vi "期末11-3-2.vi"() -> ()   [LabVIEW 2014]
uses:
  <vilib>/vision/NI_Vision_Development_Module.lvlib
panel:
  in  "計數器":dbl
  out "座標和":dbl
  in  "Boolean":bool
  out "Image Out 2":T1(plugin-control)
  out "ROI":T2
  in  "紀錄中點座標和":bool
  out "填入飽和磁場分量尖點座標和 2":dbl
  in  "3. Number of Erosion":i32=10
  out "Image Out":T1(plugin-control)
  in  "紀錄電流":dbl[](array[numeric])
  in  "Tab Control 2":enum32{"座標", "座標和", "作圖"}(tab)
  out "相減結果":dbl[](array[numeric])
  out "尖點座標和":dbl[](array[numeric])
  out "分量-電流":cluster{"紀錄電流":dbl[], dbl[]}(graph)
  in  "結束實驗":bool
  in  "1. 範圍選擇":T3={"色相（H）"={0, 255}, "飽和度（S）"={0, 255}, "亮度（L）"={0, 255}} {"亮度（L）" scale=0.0..255.0; "飽和度（S）" scale=0.0..255.0; "色相（H）" scale=0.0..255.0}
  out "Number of Particles":i32
  out "output cluster":cluster{"X":dbl, "Y":dbl}
  in  "Tab Control":T4(tab)
  out "1. 顏色選取":T1(plugin-control)
  out "2. 填補空隙":T1(plugin-control)
  out "3. 移除雜點":T1(plugin-control)
  out "4. 形狀修正":T1(plugin-control)
  out "5. 選取結果":T1(plugin-control)
  out "Particle Measurements":dbl[][](array[numeric])
  out "Error Out":errorcluster
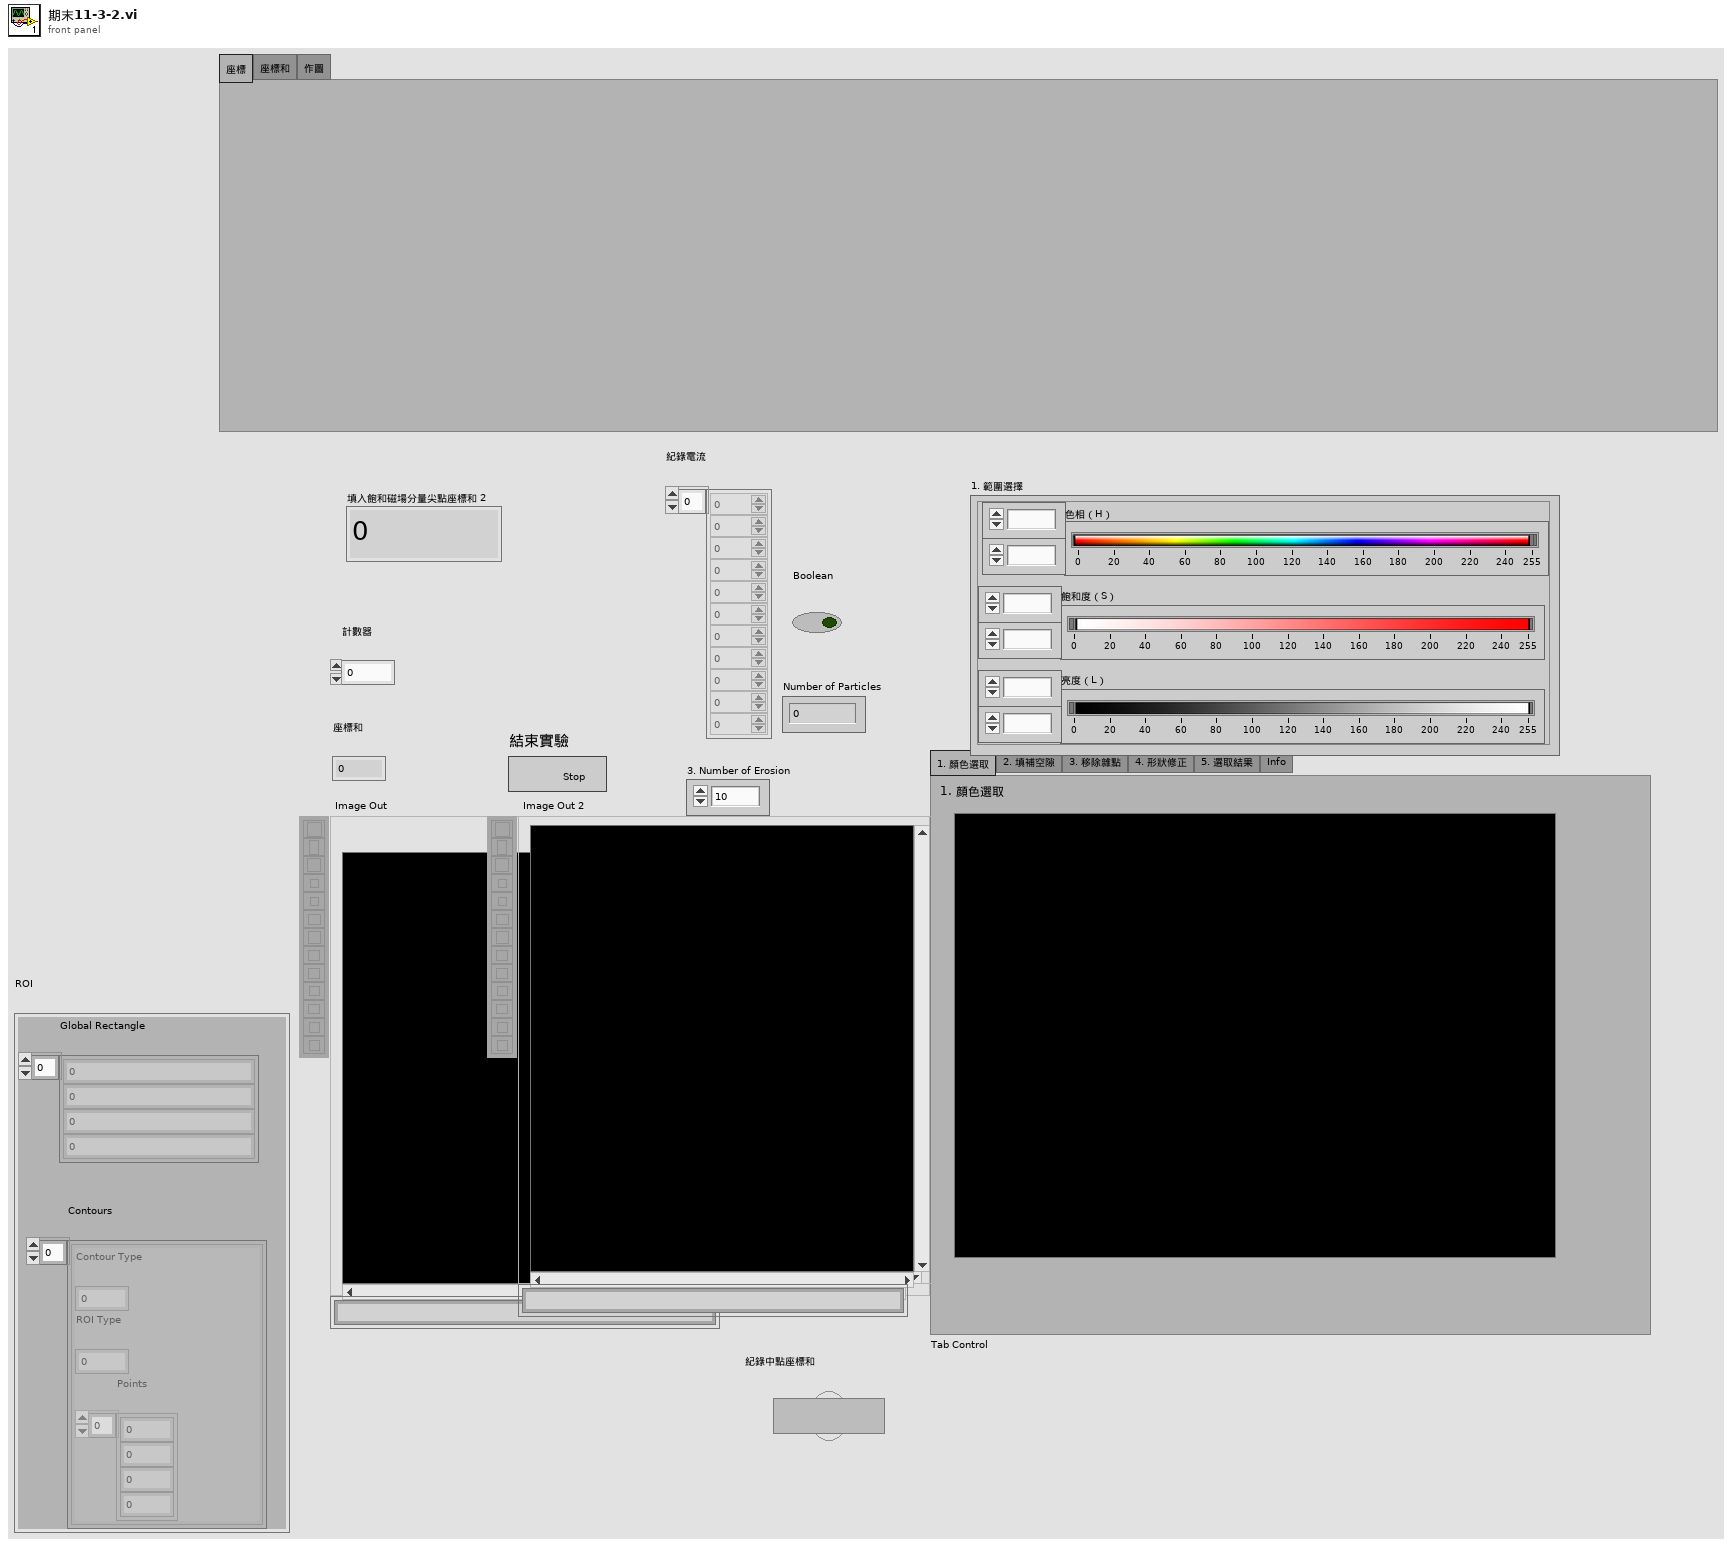
[diagram p1: front panel]
types:
  T1 = typedef "IMAQ Image.ctl" = refnum<image>
  T2 = cluster{"Global Rectangle":i32[], "Contours":cluster{"Contour Type":u32, "ROI Type":u32, "Points":i32[]}[]}
  T3 = cluster{"色相（H）":cluster{u8, u8}, "飽和度（S）":cluster{u8, u8}, "亮度（L）":cluster{u8, u8}}
  T4 = enum32{"1. 顏色選取", "2. 填補空隙", "3. 移除雜點", "4. 形狀修正", "5. 選取結果", "Info"}
  T5 = typedef "Image Type" = u32
  T6 = cluster{"Numeric":dbl, "Numeric":dbl, "Numeric":dbl, "Numeric":dbl}
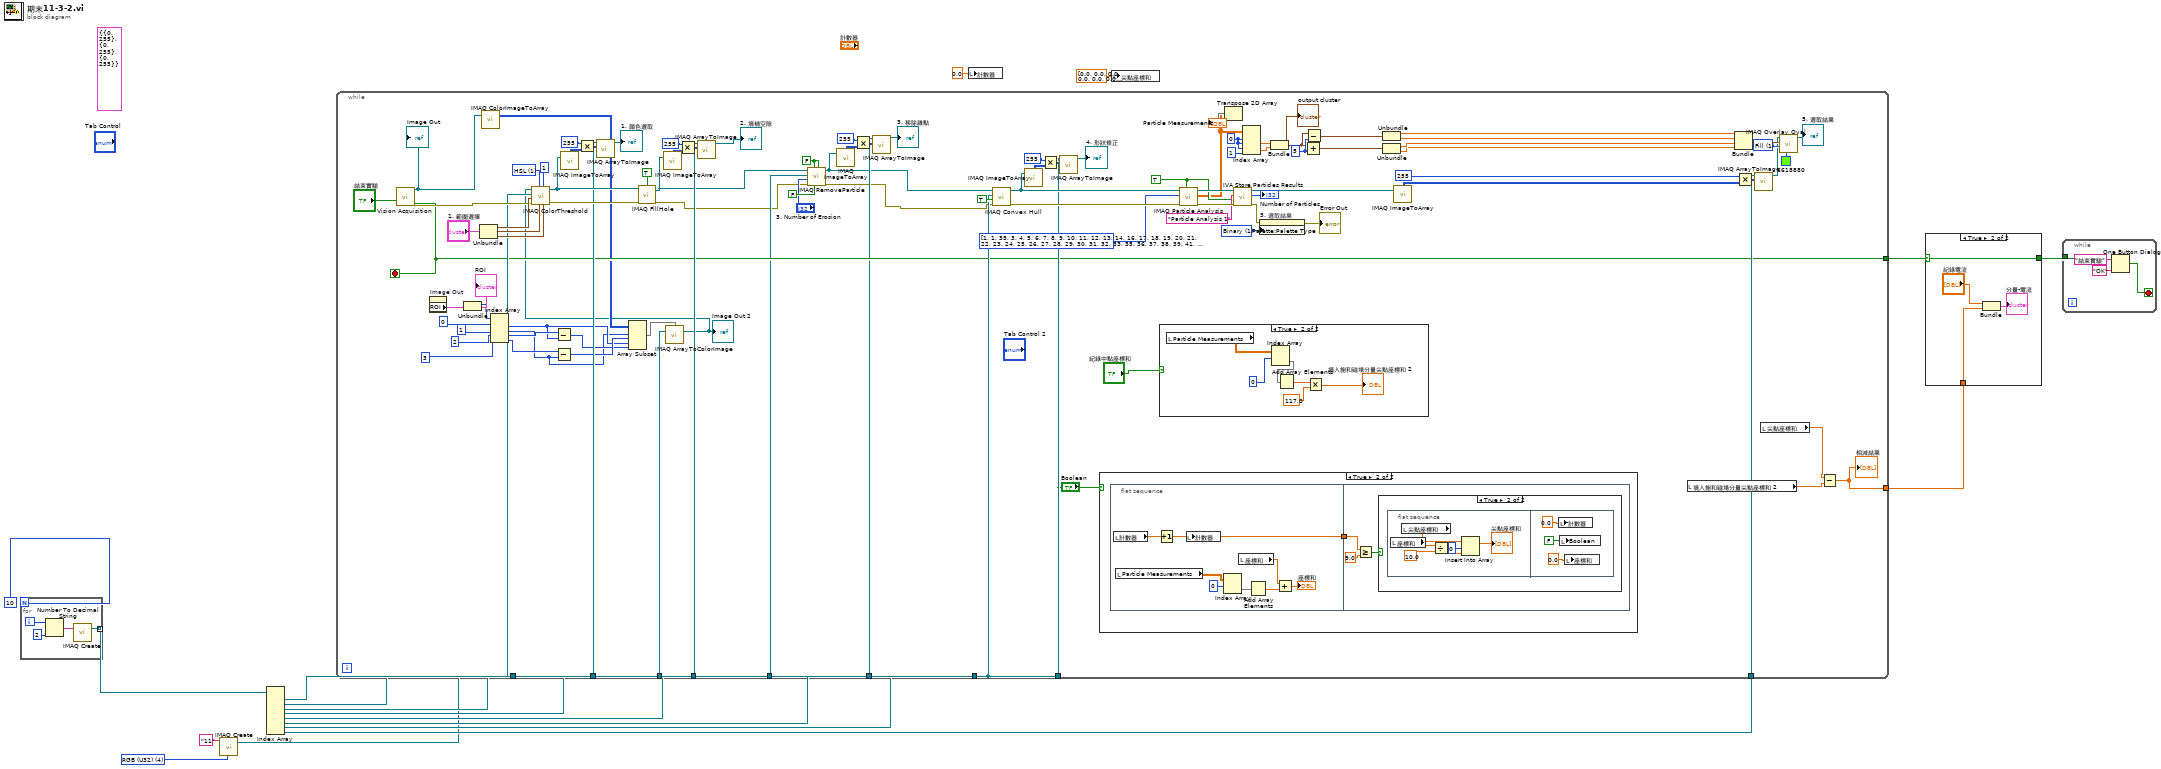
[diagram p0: block diagram]
diagram:
  w5 = T5 4 items=["Grayscale (U8)", "Grayscale (I16)", "Grayscale (SGL)", "Complex (CSG)", "RGB (U32)", "HSL (U32)", "RGB (U64)", "Grayscale (U16)"] ("Image Type")
  (unwired) T3 {"色相（H）"={0, 255}, "飽和度（S）"={0, 255}, "亮度（L）"={0, 255}} ("範圍選擇")
  n1 = for {
    N: 10 -> [_]
    tunnel: [w19] -> w18 mode=indexing
    i -> [w21]
    n2 = Number To Decimal String(number=w21, width (-)=2) -> (decimal integer string=w20:string)
    n3 = call "IMAQ Create"("Image Name"=w20) -> ("New Image"=w19:T1)  [unwired: 4 in, 1 out]
  }
  n4 = call "IMAQ Create"("Image Name"="11", "Image Type"=w5) -> ("New Image"=w6:T1)  [unwired: 3 in, 1 out]
  n5 = Index Array(array=w18) -> (element #1=w17:T1, element #2=w16:T1, element #3=w15:T1, element #4=w8:T1, element #5=w7:T1, element #6=w13:T1, element #7=w12:T1, element #8=w11:T1)  [unwired: 8 in]
  n6 = while {
    tunnel: w15 -> [w92]
    tunnel: w13 -> [w103]
    tunnel: [w103] -> _
    tunnel: w16 -> [w97]
    tunnel: w17 -> [w91]
    tunnel: w12 -> [w85]
    tunnel: w11 -> [w62]
    tunnel: [w58] -> w10
    tunnel: [w26] -> w9
    tunnel: w8 -> [w51]
    tunnel: w7 -> [w50]
    tunnel: w6 -> [w36]
    stop <- w58 stop-if-true
    w55 = FALSE ("Connectivity 4/8 (8)")
    w67 = u32 1 items=["Frame", "Fill"] ("Drawing Mode (Frame)")
    w76 = 5
    w81 = 0
    w105 = u32 1 items=["Grayscale", "Binary", "Gradient", "Rainbow", "Temperature", "User Defined"] ("Palette")
    w110 = i32[] [1, 1, 35, 3, 4, 5, 6, 7, 8, 9, 10, 11, 12, 13, 14, 16, 17, 18, 19, 20, 21, 22, 23, 24, 25, 26, 27, 28, 29, 30, 31, 32, 33, 35, 36, 37, 38, 39, 41, 42, 43, 45, 46, 48, 49, 50, 51, 53, 54, 55, 56, 58, 59, 60, 61, 62, 63, 64, 65, 66, 68, 69, 70, 71, 72, 73, 74, 75, 76, 77, 78, 79, 80, 81, 82, 83, 84, 85, 86, 87, 88] items=["Center of Mass X", "Center of Mass Y", "First Pixel X", "First Pixel Y", "Bounding Rect Left", "Bounding Rect Top", "Bounding Rect Right", "Bounding Rect Bottom", "Max Feret Diameter Start X", "Max Feret Diameter Start Y", "Max Feret Diameter End X", "Max Feret Diameter End Y", "Max Horiz. Segment Length Left", "Max Horiz. Segment Length Right", "Max Horiz. Segment Length Row", "-", "Bounding Rect Width", "Bounding Rect Height", "Bounding Rect Diagonal", "Perimeter", "Convex Hull Perimeter", "Holes' Perimeter", "Max Feret Diameter", "Equivalent Ellipse Major Axis", "Equivalent Ellipse Minor Axis", "Equivalent Ellipse Minor Axis (Feret)", "Equivalent Rect Long Side", "Equivalent Rect Short Side", "Equivalent Rect Diagonal", "Equivalent Rect Short Side (Feret)", "Average Horiz. Segment Length", "Average Vert. Segment Length", "Hydraulic Radius", "Waddel Disk Diameter", "-", "Area", "Holes' Area", "Particle & Holes' Area", "Convex Hull Area", "Image Area", "-", "Number of Holes", "Number of Horiz. Segments", "Number of Vert. Segments", "-", "Orientation", "Max Feret Diameter Orientation", "-", "% Area/Image Area", "% Area/(Particle & Holes' Area)", "Ratio of Equivalent Ellipse Axes", "Ratio of Equivalent Rect Sides", "-", "Elongation Factor", "Compactness Factor", "Heywood Circularity Factor", "Type Factor", "-", "Sum X", "Sum Y", "Sum XX", "Sum XY", "Sum YY", "Sum XXX", "Sum XXY", "Sum XYY", "Sum YYY", "-", "Moment of Inertia XX", "Moment of Inertia XY", "Moment of Inertia YY", "Moment of Inertia XXX", "Moment of Inertia XXY", "Moment of Inertia XYY", "Moment of Inertia YYY", "Norm. Moment of Inertia XX", "Norm. Moment of Inertia XY", "Norm. Moment of Inertia YY", "Norm. Moment of Inertia XXX", "Norm. Moment of Inertia XXY", "Norm. Moment of Inertia XYY", "Norm. Moment of Inertia YYY", "Hu Moment 1", "Hu Moment 2", "Hu Moment 3", "Hu Moment 4", "Hu Moment 5", "Hu Moment 6", "Hu Moment 7"] ("Pixel Measurements")
    w112 = TRUE ("Connectivity 4/8 (8)")
    w121 = u16 1 items=["RGB", "HSL", "HSV", "HSI"] ("Color Mode")
    n7 = call "Vision Acquisition"("Stop (F)"="結束實驗") -> ("Image Out"=w44:T1, "Stopped"=w58:bool, "error out"=w116:errorcluster)  [unwired: 24 in]
    "Image Out" <- w44
    n8 = property on="Image Out" class="ImageControl"() -> ("ROI"=w42:T2)  [unwired: 2 in, 2 out]
    "ROI" <- w42
    n9 = Unbundle(w42) -> ("Global Rectangle"=w41:i32[])  [unwired: 1 out]
    n10 = Unbundle("1. 範圍選擇") -> ("色相（H）"=w120:cluster{u8, u8}, "飽和度（S）"=w119:cluster{u8, u8}, "亮度（L）"=w118:cluster{u8, u8})
    n11 = call "IMAQ ColorImageToArray"("Image"=w44) -> ("Image Pixels (U32)"=w43:u32[][])  [unwired: 3 in, 2 out]
    n12 = Index Array(array=w41, index #1=0 ("index"), index #2=1 ("index"), index #3=2 ("index"), index #4=3 ("index")) -> (element #1=w31:i32, element #2=w29:i32, element #3=w34:i32, element #4=w30:i32)
    n13 = Subtract(x=w34, y=w31) -> (x-y=w32:i32)
    n14 = Subtract(x=w30, y=w29) -> (x-y=w33:i32)
    n15 = Array Subset(array=w43, index (row)=w29, length (row)=w33, index (col)=w31, length (col)=w32) -> (w35:u32[][])
    n16 = call "IMAQ ArrayToColorImage"("Image Pixels (U32)"=w35, "Image"=w36) -> ("Image Out"=w28:T1)  [unwired: 3 in, 1 out]
    "Image Out 2" <- w28
    n17 = call "IMAQ ColorThreshold"("Blue or Luma or Val or Inten Range"=w118, "Replace Value"=1, "Green or Sat Range"=w119, "Color Mode"=w121, "error in (no error)"=w116, "Red or Hue Range"=w120, "Image Dst"=w91, "Image Src"=w28) -> ("error out"=w107:errorcluster, "Image Dst Out"=w102:T1)  [unwired: 2 out]
    n18 = call "IMAQ ImageToArray"("Image"=w102) -> ("Image Pixels (U8)"=w100:u8[][])  [unwired: 3 in, 4 out]
    n19 = Multiply(x=255, y=w100) -> (x*y=w99:i32[][])
    n20 = call "IMAQ ArrayToImage"("Image Pixels (U8)"=w99, "Image"=w97) -> ("Image Out"=→"1. 顏色選取":T1)  [unwired: 8 in, 1 out]
    n21 = call "IMAQ FillHole"("error in (no error)"=w107, "Image Src"=w102, "Connectivity 4/8 (8)"=TRUE) -> ("error out"=w49:errorcluster, "Image Dst Out"=w47:T1)  [unwired: 1 in, 2 out]
    n22 = call "IMAQ ImageToArray"("Image"=w47) -> ("Image Pixels (U8)"=w95:u8[][])  [unwired: 3 in, 4 out]
    n23 = Multiply(x=255, y=w95) -> (x*y=w96:i32[][])
    n24 = call "IMAQ ArrayToImage"("Image Pixels (U8)"=w96, "Image"=w92) -> ("Image Out"=→"2. 填補空隙":T1)  [unwired: 8 in, 1 out]
    n25 = call "IMAQ RemoveParticle"("Connectivity 4/8 (8)"=w55, "Low Pass/High Pass (Low)"=FALSE, "Square/Hexa (Square)"=w55, "error in (no error)"=w49, "Number of Erosion"="3. Number of Erosion", "Image Dst"=w51, "Image Src"=w47) -> ("error out"=w48:errorcluster, "Image Dst Out"=w46:T1)  [unwired: 3 out]
    n26 = call "IMAQ ImageToArray"("Image"=w46) -> ("Image Pixels (U8)"=w45:u8[][])  [unwired: 3 in, 4 out]
    n27 = Multiply(x=255, y=w45) -> (x*y=w53:i32[][])
    n28 = call "IMAQ ArrayToImage"("Image Pixels (U8)"=w53, "Image"=w50) -> ("Image Out"=→"3. 移除雜點":T1)  [unwired: 8 in, 1 out]
    n29 = call "IMAQ Convex Hull"("error in (no error)"=w48, "Connectivity 4/8 (8)"=TRUE, "Image Dst"=w103, "Image Src"=w46) -> ("error out"=w111:errorcluster, "Image Dst Out"=w86:T1)  [unwired: 6 out]
    n30 = call "IMAQ ImageToArray"("Image"=w86) -> ("Image Pixels (U8)"=w89:u8[][])  [unwired: 3 in, 4 out]
    n31 = Multiply(x=255, y=w89) -> (x*y=w90:i32[][])
    n32 = call "IMAQ ArrayToImage"("Image Pixels (U8)"=w90, "Image"=w85) -> ("Image Out"=→"4. 形狀修正":T1)  [unwired: 8 in, 1 out]
    n33 = case shown="True" "Boolean" {
      frame False {
      }
      frame True {
        n34 = flat-sequence {
          tunnel: [w125] -> w123
          tunnel: w123 -> [w132]
          frame #0 {
            n35 = local read "計數器"() -> (w125:dbl)
            n36 = local read "Particle Measurements"() -> (w124:dbl[][])
            n37 = Increment(x=w125) -> (x+1=w126:dbl)
            n38 = local write "計數器"(w126) -> ()
            n39 = Index Array(array=w124, index (row)=0) -> (element=w130:dbl[])  [unwired: 1 in]
            n40 = local read "座標和"() -> (w129:dbl)
            n41 = Add Array Elements(numeric array=w130) -> (sum=w127:dbl)
            n42 = Add(x=w129, y=w127) -> (x+y=→"座標和":dbl)
          }
          frame #1 {
            n43 = Greater Or Equal?(x=w132, y=9.0) -> (x >= y?=w134:bool)
            n44 = case shown="True" w134 {
              frame False {
              }
              frame True {
                n45 = flat-sequence {
                  frame #0 {
                    n46 = local read "座標和"() -> (w140:dbl)
                    n47 = local read "尖點座標和"() -> (w135:dbl[])
                    n48 = Divide(x=w140, y=10.0) -> (x/y=w138:dbl)
                    n49 = Insert Into Array(array=w135, index=0, new element=w138) -> (→"尖點座標和":dbl[])
                  }
                  frame #1 {
                    n50 = local write "計數器"(0.0 ("計數器")) -> ()
                    n51 = local write "Boolean"(FALSE ("Boolean")) -> ()
                    n52 = local write "座標和"(0.0 ("座標和")) -> ()
                  }
                }
              }
            }
          }
        }
      }
    }
    n53 = case shown="True" "紀錄中點座標和" {
      frame False {
      }
      frame True {
        n54 = local read "Particle Measurements"() -> (w148:dbl[][])
        n55 = Index Array(array=w148, index (row)=0) -> (element=w147:dbl[])  [unwired: 1 in]
        n56 = Add Array Elements(numeric array=w147) -> (sum=w146:dbl)
        n57 = Multiply(x=w146, y=117.0) -> (x*y=→"填入飽和磁場分量尖點座標和 2":dbl)
      }
    }
    n58 = call "IMAQ Particle Analysis"("Connectivity 4/8 (8)"=w112, "error in (no error)"=w111, "Pixel Measurements"=w110, "Image"=w86) -> ("error out"=w115:errorcluster, "Particle Measurements (Pixels)"=w82:dbl[][], "Image Out (duplicate)"=w113:T1)  [unwired: 1 in, 4 out]
    n59 = Transpose 2D Array(2D array=w82) -> (transposed array=→"Particle Measurements":dbl[][])
    n60 = call <vilib>:"IVA Store Particles Results.vi"("error in (no error)"=w115, "Connectivity 4/8 (8)"=w112, "Step Name"="Particle Analysis 1", "Image in"=w113) -> ("error out"=w106:errorcluster, "Number of Particles"=→"Number of Particles":i32, "Image dup"=w66:T1)  [unwired: 5 out]
    n61 = Index Array(array=w82, index (row) #1=w81, index (col) #1=w81, index (row) #2=w81, index (col) #2=1) -> (element #1=w79:dbl, element #2=w78:dbl)
    n62 = property on="5. 選取結果" class="ImageControl"(error in=w106, "Palette:Palette Type"=w105) -> (error out=→"Error Out":errorcluster)  [unwired: 1 in, 1 out]
    n63 = Bundle("Numeric"=w79, "Numeric"=w78) -> (w75:cluster{"Numeric":dbl, "Numeric":dbl})  [unwired: 1 in]
    "output cluster" <- w75
    n64 = Add(x=w75, y=w76) -> (x+y=w73:cluster{"Numeric":dbl, "Numeric":dbl})
    n65 = Subtract(x=w75, y=w76) -> (x-y=w74:cluster{"Numeric":dbl, "Numeric":dbl})
    n66 = Unbundle(w74) -> ("Numeric"=w72:dbl, "Numeric"=w71:dbl)
    n67 = Unbundle(w73) -> ("Numeric"=w70:dbl, "Numeric"=w69:dbl)
    n68 = call "IMAQ ImageToArray"("Image"=w66) -> ("Image Pixels (U8)"=w63:u8[][])  [unwired: 3 in, 4 out]
    n69 = local read "填入飽和磁場分量尖點座標和 2"() -> (w27:dbl)
    n70 = Bundle("Numeric"=w72, "Numeric"=w71, "Numeric"=w70, "Numeric"=w69) -> (w68:T6)  [unwired: 1 in]
    n71 = Multiply(x=255, y=w63) -> (x*y=w64:i32[][])
    n72 = call "IMAQ ArrayToImage"("Image Pixels (U8)"=w64, "Image"=w62) -> ("Image Out"=w61:T1)  [unwired: 8 in, 1 out]
    n73 = local read "尖點座標和"() -> (w23:dbl[])
    n74 = call "IMAQ Overlay Oval"("Color"=u32 6618880, "Drawing Mode (Frame)"=w67, "Bounding Rectangle"=w68, "Image"=w61) -> ("Image Out"=→"5. 選取結果":T1)  [unwired: 6 in, 1 out]
    n75 = Subtract(x=w23, y=w27) -> (x-y=w26:dbl[])
    "相減結果" <- w26
  }
  n76 = local write "計數器"(0.0 ("計數器")) -> ()
  n77 = local write "尖點座標和"(dbl[] [0.0, 0.0, 0.0, 0.0, 0.0, 0.0, 0.0, 0.0, 0.0, 0.0, 0.0, 0.0, 0.0, 0.0, 0.0, 0.0, 0.0, 0.0, 0.0, 0.0, 0.0, 0.0, 0.0, 0.0, 0.0, 0.0, 0.0, 0.0, 0.0, 0.0, 0.0, 0.0, 0.0, 0.0, 0.0, 0.0, 0.0, 0.0, 0.0, 0.0, 0.0, 0.0, 0.0, 0.0, 0.0, 0.0, 0.0, 0.0, 0.0, 0.0, 0.0, 0.0, 0.0, 0.0, 0.0, 0.0, 0.0, 0.0, 0.0, 0.0, 0.0, 0.0, 0.0, 0.0, 0.0, 0.0, 0.0, 0.0, 0.0, 0.0, 0.0, 0.0, 0.0, 0.0, 0.0, 0.0, 0.0, 0.0, 0.0, 0.0, 0.0, 0.0, 0.0, 0.0, 0.0, 0.0, 0.0, 0.0, 0.0, 0.0, 0.0, 0.0, 0.0, 0.0, 0.0, 0.0, 0.0, 0.0, 0.0, 0.0, 0.0, 0.0, 0.0, 0.0, 0.0, 0.0, 0.0, 0.0, 0.0, 0.0, 0.0, 0.0, 0.0, 0.0, 0.0, 0.0, 0.0, 0.0, 0.0, 0.0, 0.0, 0.0, 0.0, 0.0, 0.0, 0.0, 0.0, 0.0, 0.0, 0.0, 0.0, 0.0, 0.0, 0.0, 0.0, 0.0, 0.0, 0.0, 0.0, 0.0, 0.0, 0.0, 0.0, 0.0, 0.0, 0.0, 0.0, 0.0, 0.0, 0.0, 0.0, 0.0, 0.0, 0.0, 0.0, 0.0, 0.0, 0.0, 0.0, 0.0, 0.0, 0.0, 0.0, 0.0, 0.0, 0.0, 0.0, 0.0, 0.0, 0.0, 0.0, 0.0, 0.0, 0.0, 0.0, 0.0, 0.0, 0.0, 0.0, 0.0, 0.0, 0.0, 0.0, 0.0, 0.0, 0.0, 0.0, 0.0, 0.0, 0.0, 0.0, 0.0, 0.0, 0.0, 0.0, 0.0, 0.0, 0.0, 0.0, 0.0, 0.0, 0.0, 0.0, 0.0, 0.0, 0.0, 0.0, 0.0, 0.0, 0.0, 0.0, 0.0, 0.0, 0.0, 0.0, 0.0, 0.0, 0.0, 0.0, 0.0, 0.0, 0.0, 0.0, 0.0, 0.0, 0.0, 0.0, 0.0, 0.0, 0.0, 0.0, 0.0, 0.0, 0.0, 0.0, 0.0, 0.0, 0.0, 0.0, 0.0, 0.0, 0.0, 0.0, 0.0, 0.0, 0.0, 0.0, 0.0, 0.0, 0.0, 0.0, 0.0, 0.0, 0.0, 0.0, 0.0, 0.0, 0.0, 0.0, 0.0, 0.0, 0.0, 0.0, 0.0, 0.0, 0.0, 0.0, 0.0, 0.0, 0.0, 0.0, 0.0, 0.0, 0.0, 0.0, 0.0, 0.0, 0.0, 0.0, 0.0, 0.0, 0.0, 0.0, 0.0, 0.0, 0.0, 0.0, 0.0, 0.0, 0.0, 0.0, 0.0, 0.0, 0.0, 0.0, 0.0, 0.0, 0.0, 0.0, 0.0, 0.0, 0.0, 0.0, 0.0, 0.0, 0.0, 0.0, 0.0, 0.0, 0.0, 0.0, 0.0, 0.0, 0.0, 0.0, 0.0, 0.0, 0.0, 0.0, 0.0, 0.0, 0.0, 0.0, 0.0, 0.0, 0.0, 0.0, 0.0, 0.0, 0.0, 0.0, 0.0, 0.0, 0.0, 0.0, 0.0, 0.0, 0.0, 0.0, 0.0, 0.0, 0.0, 0.0, 0.0, 0.0, 0.0, 0.0, 0.0, 0.0, 0.0, 0.0, 0.0, 0.0, 0.0, 0.0, 0.0, 0.0, 0.0, 0.0, 0.0, 0.0, 0.0, 0.0, 0.0, 0.0, 0.0, 0.0, 0.0, 0.0, 0.0, 0.0, 0.0, 0.0, 0.0, 0.0, 0.0, 0.0, 0.0, 0.0, 0.0, 0.0, 0.0, 0.0, 0.0, 0.0, 0.0, 0.0, 0.0, 0.0, 0.0, 0.0, 0.0, 0.0, 0.0, 0.0, 0.0, 0.0, 0.0, 0.0, 0.0, 0.0, 0.0, 0.0, 0.0, 0.0, 0.0, 0.0, 0.0, 0.0, 0.0, 0.0, 0.0, 0.0, 0.0, 0.0, 0.0, 0.0, 0.0, 0.0, 0.0, 0.0, 0.0, 0.0, 0.0, 0.0, 0.0, 0.0, 0.0, 0.0, 0.0, 0.0, 0.0, 0.0, 0.0, 0.0, 0.0, 0.0, 0.0, 0.0, 0.0, 0.0, 0.0, 0.0, 0.0, 0.0, 0.0, 0.0, 0.0, 0.0, 0.0, 0.0, 0.0, 0.0, 0.0, 0.0, 0.0, 0.0, 0.0, 0.0, 0.0, 0.0, 0.0, 0.0, 0.0, 0.0, 0.0, 0.0, 0.0, 0.0, 0.0, 0.0, 0.0, 0.0, 0.0, 0.0, 0.0, 0.0, 0.0, 0.0, 0.0, 0.0, 0.0, 0.0, 0.0, 0.0, 0.0, 0.0, 0.0, 0.0, 0.0, 0.0, 0.0, 0.0, 0.0, 0.0, 0.0, 0.0, 0.0, 0.0, 0.0, 0.0, 0.0, 0.0, 0.0, 0.0, 0.0, 0.0, 0.0, 0.0, 0.0, 0.0, 0.0, 0.0, 0.0, 0.0, 0.0, 0.0, 0.0, 0.0, 0.0, 0.0, 0.0, 0.0, 0.0, 0.0, 0.0, 0.0, 0.0, 0.0, 0.0, 0.0, 0.0, 0.0, 0.0, 0.0, 0.0, 0.0, 0.0, 0.0, 0.0, 0.0, 0.0, 0.0, 0.0, 0.0, 0.0, 0.0, 0.0, 0.0, 0.0, 0.0, 0.0, 0.0, 0.0, 0.0, 0.0, 0.0, 0.0, 0.0, 0.0, 0.0, 0.0, 0.0, 0.0, 0.0, 0.0, 0.0, 0.0, 0.0, 0.0, 0.0, 0.0, 0.0, 0.0, 0.0, 0.0, 0.0, 0.0, 0.0, 0.0, 0.0, 0.0, 0.0, 0.0, 0.0, 0.0, 0.0, 0.0, 0.0, 0.0, 0.0, 0.0, 0.0, 0.0, 0.0, 0.0, 0.0, 0.0, 0.0, 0.0, 0.0, 0.0, 0.0, 0.0, 0.0, 0.0, 0.0, 0.0, 0.0, 0.0, 0.0, 0.0, 0.0, 0.0, 0.0, 0.0, 0.0, 0.0, 0.0, 0.0, 0.0, 0.0, 0.0, 0.0, 0.0, 0.0, 0.0, 0.0, 0.0, 0.0, 0.0, 0.0, 0.0, 0.0, 0.0, 0.0, 0.0, 0.0, 0.0, 0.0, 0.0, 0.0, 0.0, 0.0, 0.0, 0.0, 0.0, 0.0, 0.0, 0.0, 0.0, 0.0, 0.0, 0.0, 0.0, 0.0, 0.0, 0.0, 0.0, 0.0, 0.0, 0.0, 0.0, 0.0, 0.0, 0.0, 0.0, 0.0, 0.0, 0.0] ("尖點座標和")) -> ()
  n78 = case shown="True" w10 {
    selector: w10 -> [w150 w154]
    tunnel: [w150 w154] -> w3
    tunnel: w9 -> [_ w153]
    frame False {
    }
    frame True {
      n79 = Bundle("紀錄電流"="紀錄電流", w153) -> (→"分量-電流":cluster{"紀錄電流":dbl[], dbl[]})  [unwired: 1 in]
    }
  }
  n80 = while {
    tunnel: w3 -> [_]
    stop <- w157 stop-if-true
    n81 = One Button Dialog(message="結束實驗", button name ("OK")="OK") -> (true=w157:bool)
  }
